vi "数字量输入配置.vi"() -> ()   [LabVIEW 2010] (continued)
              n4462 = local write "单选_第14路"(w132) -> ()
              n4463 = local write "单选_第15路"(w132) -> ()
              n4464 = local write "单选_第16路"(w132) -> ()
              n4465 = local write "单选_第17路"(w132) -> ()
              n4466 = local write "单选_第18路"(w132) -> ()
              n4467 = local write "单选_第19路"(w132) -> ()
              n4468 = local write "单选_第20路"(w132) -> ()
              n4469 = local write "单选_第21路"(w132) -> ()
              n4470 = local write "单选_第22路"(w132) -> ()
              n4471 = local write "单选_第23路"(w132) -> ()
              n4472 = local write "单选_第24路"(w132) -> ()
              n4473 = local write "单选_第25路"(w132) -> ()
              n4474 = local write "单选_第26路"(w132) -> ()
              n4475 = local write "单选_第27路"(w132) -> ()
              n4476 = local write "单选_第28路"(w132) -> ()
              n4477 = local write "单选_第29路"(w132) -> ()
              n4478 = local write "单选_第30路"(w132) -> ()
              n4479 = local write "单选_第31路"(w132) -> ()
              n4480 = local write "单选_第32路"(w132) -> ()
              n4481 = local write "单选_第33路"(w132) -> ()
              n4482 = local write "单选_第34路"(w132) -> ()
              n4483 = local write "单选_第35路"(w132) -> ()
              n4484 = local write "单选_第36路"(w132) -> ()
              n4485 = local write "单选_第37路"(w132) -> ()
              n4486 = local write "单选_第38路"(w132) -> ()
              n4487 = local write "单选_第39路"(w132) -> ()
              n4488 = local write "单选_第40路"(w132) -> ()
              n4489 = local write "单选_第41路"(w132) -> ()
              n4490 = local write "单选_第42路"(w132) -> ()
              n4491 = local write "单选_第43路"(w132) -> ()
              n4492 = local write "单选_第44路"(w132) -> ()
              n4493 = local write "单选_第45路"(w132) -> ()
              n4494 = local write "单选_第46路"(w132) -> ()
              n4495 = local write "单选_第47路"(w132) -> ()
              n4496 = local write "单选_第48路"(w132) -> ()
              n4497 = local write "单选_第49路"(w132) -> ()
              n4498 = local write "单选_第50路"(w132) -> ()
              n4499 = local write "单选_第51路"(w133) -> ()
              n4500 = local write "单选_第52路"(w133) -> ()
              n4501 = local write "单选_第53路"(w133) -> ()
              n4502 = local write "单选_第54路"(w133) -> ()
              n4503 = local write "单选_第55路"(w133) -> ()
              n4504 = local write "单选_第56路"(w133) -> ()
              n4505 = local write "单选_第57路"(w133) -> ()
              n4506 = local write "单选_第58路"(w133) -> ()
              n4507 = local write "单选_第59路"(w133) -> ()
              n4508 = local write "单选_第60路"(w133) -> ()
              n4509 = local write "单选_第61路"(w133) -> ()
              n4510 = local write "单选_第62路"(w133) -> ()
              n4511 = local write "单选_第63路"(w133) -> ()
              n4512 = local write "单选_第64路"(w133) -> ()
              n4513 = local write "单选_第71路"(w133) -> ()
              n4514 = local write "单选_第79路"(w133) -> ()
              n4515 = local write "单选_第65路"(w133) -> ()
              n4516 = local write "单选_第66路"(w133) -> ()
              n4517 = local write "单选_第67路"(w133) -> ()
              n4518 = local write "单选_第68路"(w133) -> ()
              n4519 = local write "单选_第69路"(w133) -> ()
              n4520 = local write "单选_第70路"(w133) -> ()
              n4521 = local write "单选_第72路"(w133) -> ()
              n4522 = local write "单选_第73路"(w133) -> ()
              n4523 = local write "单选_第74路"(w133) -> ()
              n4524 = local write "单选_第75路"(w133) -> ()
              n4525 = local write "单选_第76路"(w133) -> ()
              n4526 = local write "单选_第77路"(w133) -> ()
              n4527 = local write "单选_第78路"(w133) -> ()
              n4528 = local write "单选_第80路"(w133) -> ()
            }
            frame 51 {
              w134 = TRUE
              w135 = FALSE ("单选_第41路")
              n4529 = local write "单选_第1路"(w134) -> ()
              n4530 = local write "单选_第2路"(w134) -> ()
              n4531 = local write "单选_第3路"(w134) -> ()
              n4532 = local write "单选_第4路"(w134) -> ()
              n4533 = local write "单选_第5路"(w134) -> ()
              n4534 = local write "单选_第6路"(w134) -> ()
              n4535 = local write "单选_第7路"(w134) -> ()
              n4536 = local write "单选_第8路"(w134) -> ()
              n4537 = local write "单选_第9路"(w134) -> ()
              n4538 = local write "单选_第10路"(w134) -> ()
              n4539 = local write "单选_第11路"(w134) -> ()
              n4540 = local write "单选_第12路"(w134) -> ()
              n4541 = local write "单选_第13路"(w134) -> ()
              n4542 = local write "单选_第14路"(w134) -> ()
              n4543 = local write "单选_第15路"(w134) -> ()
              n4544 = local write "单选_第16路"(w134) -> ()
              n4545 = local write "单选_第17路"(w134) -> ()
              n4546 = local write "单选_第18路"(w134) -> ()
              n4547 = local write "单选_第19路"(w134) -> ()
              n4548 = local write "单选_第20路"(w134) -> ()
              n4549 = local write "单选_第21路"(w134) -> ()
              n4550 = local write "单选_第22路"(w134) -> ()
              n4551 = local write "单选_第23路"(w134) -> ()
              n4552 = local write "单选_第24路"(w134) -> ()
              n4553 = local write "单选_第25路"(w134) -> ()
              n4554 = local write "单选_第26路"(w134) -> ()
              n4555 = local write "单选_第27路"(w134) -> ()
              n4556 = local write "单选_第28路"(w134) -> ()
              n4557 = local write "单选_第29路"(w134) -> ()
              n4558 = local write "单选_第30路"(w134) -> ()
              n4559 = local write "单选_第31路"(w134) -> ()
              n4560 = local write "单选_第32路"(w134) -> ()
              n4561 = local write "单选_第33路"(w134) -> ()
              n4562 = local write "单选_第34路"(w134) -> ()
              n4563 = local write "单选_第35路"(w134) -> ()
              n4564 = local write "单选_第36路"(w134) -> ()
              n4565 = local write "单选_第37路"(w134) -> ()
              n4566 = local write "单选_第38路"(w134) -> ()
              n4567 = local write "单选_第39路"(w134) -> ()
              n4568 = local write "单选_第40路"(w134) -> ()
              n4569 = local write "单选_第41路"(w134) -> ()
              n4570 = local write "单选_第42路"(w134) -> ()
              n4571 = local write "单选_第43路"(w134) -> ()
              n4572 = local write "单选_第44路"(w134) -> ()
              n4573 = local write "单选_第45路"(w134) -> ()
              n4574 = local write "单选_第46路"(w134) -> ()
              n4575 = local write "单选_第47路"(w134) -> ()
              n4576 = local write "单选_第48路"(w134) -> ()
              n4577 = local write "单选_第49路"(w134) -> ()
              n4578 = local write "单选_第50路"(w134) -> ()
              n4579 = local write "单选_第51路"(w134) -> ()
              n4580 = local write "单选_第52路"(w135) -> ()
              n4581 = local write "单选_第53路"(w135) -> ()
              n4582 = local write "单选_第54路"(w135) -> ()
              n4583 = local write "单选_第55路"(w135) -> ()
              n4584 = local write "单选_第56路"(w135) -> ()
              n4585 = local write "单选_第57路"(w135) -> ()
              n4586 = local write "单选_第58路"(w135) -> ()
              n4587 = local write "单选_第59路"(w135) -> ()
              n4588 = local write "单选_第60路"(w135) -> ()
              n4589 = local write "单选_第61路"(w135) -> ()
              n4590 = local write "单选_第62路"(w135) -> ()
              n4591 = local write "单选_第63路"(w135) -> ()
              n4592 = local write "单选_第64路"(w135) -> ()
              n4593 = local write "单选_第71路"(w135) -> ()
              n4594 = local write "单选_第79路"(w135) -> ()
              n4595 = local write "单选_第65路"(w135) -> ()
              n4596 = local write "单选_第66路"(w135) -> ()
              n4597 = local write "单选_第67路"(w135) -> ()
              n4598 = local write "单选_第68路"(w135) -> ()
              n4599 = local write "单选_第69路"(w135) -> ()
              n4600 = local write "单选_第70路"(w135) -> ()
              n4601 = local write "单选_第72路"(w135) -> ()
              n4602 = local write "单选_第73路"(w135) -> ()
              n4603 = local write "单选_第74路"(w135) -> ()
              n4604 = local write "单选_第75路"(w135) -> ()
              n4605 = local write "单选_第76路"(w135) -> ()
              n4606 = local write "单选_第77路"(w135) -> ()
              n4607 = local write "单选_第78路"(w135) -> ()
              n4608 = local write "单选_第80路"(w135) -> ()
            }
            frame 52 {
              w136 = TRUE
              w137 = FALSE ("单选_第41路")
              n4609 = local write "单选_第1路"(w136) -> ()
              n4610 = local write "单选_第2路"(w136) -> ()
              n4611 = local write "单选_第3路"(w136) -> ()
              n4612 = local write "单选_第4路"(w136) -> ()
              n4613 = local write "单选_第5路"(w136) -> ()
              n4614 = local write "单选_第6路"(w136) -> ()
              n4615 = local write "单选_第7路"(w136) -> ()
              n4616 = local write "单选_第8路"(w136) -> ()
              n4617 = local write "单选_第9路"(w136) -> ()
              n4618 = local write "单选_第10路"(w136) -> ()
              n4619 = local write "单选_第11路"(w136) -> ()
              n4620 = local write "单选_第12路"(w136) -> ()
              n4621 = local write "单选_第13路"(w136) -> ()
              n4622 = local write "单选_第14路"(w136) -> ()
              n4623 = local write "单选_第15路"(w136) -> ()
              n4624 = local write "单选_第16路"(w136) -> ()
              n4625 = local write "单选_第17路"(w136) -> ()
              n4626 = local write "单选_第18路"(w136) -> ()
              n4627 = local write "单选_第19路"(w136) -> ()
              n4628 = local write "单选_第20路"(w136) -> ()
              n4629 = local write "单选_第21路"(w136) -> ()
              n4630 = local write "单选_第22路"(w136) -> ()
              n4631 = local write "单选_第23路"(w136) -> ()
              n4632 = local write "单选_第24路"(w136) -> ()
              n4633 = local write "单选_第25路"(w136) -> ()
              n4634 = local write "单选_第26路"(w136) -> ()
              n4635 = local write "单选_第27路"(w136) -> ()
              n4636 = local write "单选_第28路"(w136) -> ()
              n4637 = local write "单选_第29路"(w136) -> ()
              n4638 = local write "单选_第30路"(w136) -> ()
              n4639 = local write "单选_第31路"(w136) -> ()
              n4640 = local write "单选_第32路"(w136) -> ()
              n4641 = local write "单选_第33路"(w136) -> ()
              n4642 = local write "单选_第34路"(w136) -> ()
              n4643 = local write "单选_第35路"(w136) -> ()
              n4644 = local write "单选_第36路"(w136) -> ()
              n4645 = local write "单选_第37路"(w136) -> ()
              n4646 = local write "单选_第38路"(w136) -> ()
              n4647 = local write "单选_第39路"(w136) -> ()
              n4648 = local write "单选_第40路"(w136) -> ()
              n4649 = local write "单选_第41路"(w136) -> ()
              n4650 = local write "单选_第42路"(w136) -> ()
              n4651 = local write "单选_第43路"(w136) -> ()
              n4652 = local write "单选_第44路"(w136) -> ()
              n4653 = local write "单选_第45路"(w136) -> ()
              n4654 = local write "单选_第46路"(w136) -> ()
              n4655 = local write "单选_第47路"(w136) -> ()
              n4656 = local write "单选_第48路"(w136) -> ()
              n4657 = local write "单选_第49路"(w136) -> ()
              n4658 = local write "单选_第50路"(w136) -> ()
              n4659 = local write "单选_第51路"(w136) -> ()
              n4660 = local write "单选_第52路"(w136) -> ()
              n4661 = local write "单选_第53路"(w137) -> ()
              n4662 = local write "单选_第54路"(w137) -> ()
              n4663 = local write "单选_第55路"(w137) -> ()
              n4664 = local write "单选_第56路"(w137) -> ()
              n4665 = local write "单选_第57路"(w137) -> ()
              n4666 = local write "单选_第58路"(w137) -> ()
              n4667 = local write "单选_第59路"(w137) -> ()
              n4668 = local write "单选_第60路"(w137) -> ()
              n4669 = local write "单选_第61路"(w137) -> ()
              n4670 = local write "单选_第62路"(w137) -> ()
              n4671 = local write "单选_第63路"(w137) -> ()
              n4672 = local write "单选_第64路"(w137) -> ()
              n4673 = local write "单选_第71路"(w137) -> ()
              n4674 = local write "单选_第79路"(w137) -> ()
              n4675 = local write "单选_第65路"(w137) -> ()
              n4676 = local write "单选_第66路"(w137) -> ()
              n4677 = local write "单选_第67路"(w137) -> ()
              n4678 = local write "单选_第68路"(w137) -> ()
              n4679 = local write "单选_第69路"(w137) -> ()
              n4680 = local write "单选_第70路"(w137) -> ()
              n4681 = local write "单选_第72路"(w137) -> ()
              n4682 = local write "单选_第73路"(w137) -> ()
              n4683 = local write "单选_第74路"(w137) -> ()
              n4684 = local write "单选_第75路"(w137) -> ()
              n4685 = local write "单选_第76路"(w137) -> ()
              n4686 = local write "单选_第77路"(w137) -> ()
              n4687 = local write "单选_第78路"(w137) -> ()
              n4688 = local write "单选_第80路"(w137) -> ()
            }
            frame 53 {
              w138 = TRUE
              w139 = FALSE ("单选_第41路")
              n4689 = local write "单选_第1路"(w138) -> ()
              n4690 = local write "单选_第2路"(w138) -> ()
              n4691 = local write "单选_第3路"(w138) -> ()
              n4692 = local write "单选_第4路"(w138) -> ()
              n4693 = local write "单选_第5路"(w138) -> ()
              n4694 = local write "单选_第6路"(w138) -> ()
              n4695 = local write "单选_第7路"(w138) -> ()
              n4696 = local write "单选_第8路"(w138) -> ()
              n4697 = local write "单选_第9路"(w138) -> ()
              n4698 = local write "单选_第10路"(w138) -> ()
              n4699 = local write "单选_第11路"(w138) -> ()
              n4700 = local write "单选_第12路"(w138) -> ()
              n4701 = local write "单选_第13路"(w138) -> ()
              n4702 = local write "单选_第14路"(w138) -> ()
              n4703 = local write "单选_第15路"(w138) -> ()
              n4704 = local write "单选_第16路"(w138) -> ()
              n4705 = local write "单选_第17路"(w138) -> ()
              n4706 = local write "单选_第18路"(w138) -> ()
              n4707 = local write "单选_第19路"(w138) -> ()
              n4708 = local write "单选_第20路"(w138) -> ()
              n4709 = local write "单选_第21路"(w138) -> ()
              n4710 = local write "单选_第22路"(w138) -> ()
              n4711 = local write "单选_第23路"(w138) -> ()
              n4712 = local write "单选_第24路"(w138) -> ()
              n4713 = local write "单选_第25路"(w138) -> ()
              n4714 = local write "单选_第26路"(w138) -> ()
              n4715 = local write "单选_第27路"(w138) -> ()
              n4716 = local write "单选_第28路"(w138) -> ()
              n4717 = local write "单选_第29路"(w138) -> ()
              n4718 = local write "单选_第30路"(w138) -> ()
              n4719 = local write "单选_第31路"(w138) -> ()
              n4720 = local write "单选_第32路"(w138) -> ()
              n4721 = local write "单选_第33路"(w138) -> ()
              n4722 = local write "单选_第34路"(w138) -> ()
              n4723 = local write "单选_第35路"(w138) -> ()
              n4724 = local write "单选_第36路"(w138) -> ()
              n4725 = local write "单选_第37路"(w138) -> ()
              n4726 = local write "单选_第38路"(w138) -> ()
              n4727 = local write "单选_第39路"(w138) -> ()
              n4728 = local write "单选_第40路"(w138) -> ()
              n4729 = local write "单选_第41路"(w138) -> ()
              n4730 = local write "单选_第42路"(w138) -> ()
              n4731 = local write "单选_第43路"(w138) -> ()
              n4732 = local write "单选_第44路"(w138) -> ()
              n4733 = local write "单选_第45路"(w138) -> ()
              n4734 = local write "单选_第46路"(w138) -> ()
              n4735 = local write "单选_第47路"(w138) -> ()
              n4736 = local write "单选_第48路"(w138) -> ()
              n4737 = local write "单选_第49路"(w138) -> ()
              n4738 = local write "单选_第50路"(w138) -> ()
              n4739 = local write "单选_第51路"(w138) -> ()
              n4740 = local write "单选_第52路"(w138) -> ()
              n4741 = local write "单选_第53路"(w138) -> ()
              n4742 = local write "单选_第54路"(w139) -> ()
              n4743 = local write "单选_第55路"(w139) -> ()
              n4744 = local write "单选_第56路"(w139) -> ()
              n4745 = local write "单选_第57路"(w139) -> ()
              n4746 = local write "单选_第58路"(w139) -> ()
              n4747 = local write "单选_第59路"(w139) -> ()
              n4748 = local write "单选_第60路"(w139) -> ()
              n4749 = local write "单选_第61路"(w139) -> ()
              n4750 = local write "单选_第62路"(w139) -> ()
              n4751 = local write "单选_第63路"(w139) -> ()
              n4752 = local write "单选_第64路"(w139) -> ()
              n4753 = local write "单选_第71路"(w139) -> ()
              n4754 = local write "单选_第79路"(w139) -> ()
              n4755 = local write "单选_第65路"(w139) -> ()
              n4756 = local write "单选_第66路"(w139) -> ()
              n4757 = local write "单选_第67路"(w139) -> ()
              n4758 = local write "单选_第68路"(w139) -> ()
              n4759 = local write "单选_第69路"(w139) -> ()
              n4760 = local write "单选_第70路"(w139) -> ()
              n4761 = local write "单选_第72路"(w139) -> ()
              n4762 = local write "单选_第73路"(w139) -> ()
              n4763 = local write "单选_第74路"(w139) -> ()
              n4764 = local write "单选_第75路"(w139) -> ()
              n4765 = local write "单选_第76路"(w139) -> ()
              n4766 = local write "单选_第77路"(w139) -> ()
              n4767 = local write "单选_第78路"(w139) -> ()
              n4768 = local write "单选_第80路"(w139) -> ()
            }
            frame 54 {
              w140 = TRUE
              w141 = FALSE ("单选_第41路")
              n4769 = local write "单选_第1路"(w140) -> ()
              n4770 = local write "单选_第2路"(w140) -> ()
              n4771 = local write "单选_第3路"(w140) -> ()
              n4772 = local write "单选_第4路"(w140) -> ()
              n4773 = local write "单选_第5路"(w140) -> ()
              n4774 = local write "单选_第6路"(w140) -> ()
              n4775 = local write "单选_第7路"(w140) -> ()
              n4776 = local write "单选_第8路"(w140) -> ()
              n4777 = local write "单选_第9路"(w140) -> ()
              n4778 = local write "单选_第10路"(w140) -> ()
              n4779 = local write "单选_第11路"(w140) -> ()
              n4780 = local write "单选_第12路"(w140) -> ()
              n4781 = local write "单选_第13路"(w140) -> ()
              n4782 = local write "单选_第14路"(w140) -> ()
              n4783 = local write "单选_第15路"(w140) -> ()
              n4784 = local write "单选_第16路"(w140) -> ()
              n4785 = local write "单选_第17路"(w140) -> ()
              n4786 = local write "单选_第18路"(w140) -> ()
              n4787 = local write "单选_第19路"(w140) -> ()
              n4788 = local write "单选_第20路"(w140) -> ()
              n4789 = local write "单选_第21路"(w140) -> ()
              n4790 = local write "单选_第22路"(w140) -> ()
              n4791 = local write "单选_第23路"(w140) -> ()
              n4792 = local write "单选_第24路"(w140) -> ()
              n4793 = local write "单选_第25路"(w140) -> ()
              n4794 = local write "单选_第26路"(w140) -> ()
              n4795 = local write "单选_第27路"(w140) -> ()
              n4796 = local write "单选_第28路"(w140) -> ()
              n4797 = local write "单选_第29路"(w140) -> ()
              n4798 = local write "单选_第30路"(w140) -> ()
              n4799 = local write "单选_第31路"(w140) -> ()
              n4800 = local write "单选_第32路"(w140) -> ()
              n4801 = local write "单选_第33路"(w140) -> ()
              n4802 = local write "单选_第34路"(w140) -> ()
              n4803 = local write "单选_第35路"(w140) -> ()
              n4804 = local write "单选_第36路"(w140) -> ()
              n4805 = local write "单选_第37路"(w140) -> ()
              n4806 = local write "单选_第38路"(w140) -> ()
              n4807 = local write "单选_第39路"(w140) -> ()
              n4808 = local write "单选_第40路"(w140) -> ()
              n4809 = local write "单选_第41路"(w140) -> ()
              n4810 = local write "单选_第42路"(w140) -> ()
              n4811 = local write "单选_第43路"(w140) -> ()
              n4812 = local write "单选_第44路"(w140) -> ()
              n4813 = local write "单选_第45路"(w140) -> ()
              n4814 = local write "单选_第46路"(w140) -> ()
              n4815 = local write "单选_第47路"(w140) -> ()
              n4816 = local write "单选_第48路"(w140) -> ()
              n4817 = local write "单选_第49路"(w140) -> ()
              n4818 = local write "单选_第50路"(w140) -> ()
              n4819 = local write "单选_第51路"(w140) -> ()
              n4820 = local write "单选_第52路"(w140) -> ()
              n4821 = local write "单选_第53路"(w140) -> ()
              n4822 = local write "单选_第54路"(w140) -> ()
              n4823 = local write "单选_第55路"(w141) -> ()
              n4824 = local write "单选_第56路"(w141) -> ()
              n4825 = local write "单选_第57路"(w141) -> ()
              n4826 = local write "单选_第58路"(w141) -> ()
              n4827 = local write "单选_第59路"(w141) -> ()
              n4828 = local write "单选_第60路"(w141) -> ()
              n4829 = local write "单选_第61路"(w141) -> ()
              n4830 = local write "单选_第62路"(w141) -> ()
              n4831 = local write "单选_第63路"(w141) -> ()
              n4832 = local write "单选_第64路"(w141) -> ()
              n4833 = local write "单选_第71路"(w141) -> ()
              n4834 = local write "单选_第79路"(w141) -> ()
              n4835 = local write "单选_第65路"(w141) -> ()
              n4836 = local write "单选_第66路"(w141) -> ()
              n4837 = local write "单选_第67路"(w141) -> ()
              n4838 = local write "单选_第68路"(w141) -> ()
              n4839 = local write "单选_第69路"(w141) -> ()
              n4840 = local write "单选_第70路"(w141) -> ()
              n4841 = local write "单选_第72路"(w141) -> ()
              n4842 = local write "单选_第73路"(w141) -> ()
              n4843 = local write "单选_第74路"(w141) -> ()
              n4844 = local write "单选_第75路"(w141) -> ()
              n4845 = local write "单选_第76路"(w141) -> ()
              n4846 = local write "单选_第77路"(w141) -> ()
              n4847 = local write "单选_第78路"(w141) -> ()
              n4848 = local write "单选_第80路"(w141) -> ()
            }
            frame 55 {
              w142 = TRUE
              w143 = FALSE ("单选_第41路")
              n4849 = local write "单选_第1路"(w142) -> ()
              n4850 = local write "单选_第2路"(w142) -> ()
              n4851 = local write "单选_第3路"(w142) -> ()
              n4852 = local write "单选_第4路"(w142) -> ()
              n4853 = local write "单选_第5路"(w142) -> ()
              n4854 = local write "单选_第6路"(w142) -> ()
              n4855 = local write "单选_第7路"(w142) -> ()
              n4856 = local write "单选_第8路"(w142) -> ()
              n4857 = local write "单选_第9路"(w142) -> ()
              n4858 = local write "单选_第10路"(w142) -> ()
              n4859 = local write "单选_第11路"(w142) -> ()
              n4860 = local write "单选_第12路"(w142) -> ()
              n4861 = local write "单选_第13路"(w142) -> ()
              n4862 = local write "单选_第14路"(w142) -> ()
              n4863 = local write "单选_第15路"(w142) -> ()
              n4864 = local write "单选_第16路"(w142) -> ()
              n4865 = local write "单选_第17路"(w142) -> ()
              n4866 = local write "单选_第18路"(w142) -> ()
              n4867 = local write "单选_第19路"(w142) -> ()
              n4868 = local write "单选_第20路"(w142) -> ()
              n4869 = local write "单选_第21路"(w142) -> ()
              n4870 = local write "单选_第22路"(w142) -> ()
              n4871 = local write "单选_第23路"(w142) -> ()
              n4872 = local write "单选_第24路"(w142) -> ()
              n4873 = local write "单选_第25路"(w142) -> ()
              n4874 = local write "单选_第26路"(w142) -> ()
              n4875 = local write "单选_第27路"(w142) -> ()
              n4876 = local write "单选_第28路"(w142) -> ()
              n4877 = local write "单选_第29路"(w142) -> ()
              n4878 = local write "单选_第30路"(w142) -> ()
              n4879 = local write "单选_第31路"(w142) -> ()
              n4880 = local write "单选_第32路"(w142) -> ()
              n4881 = local write "单选_第33路"(w142) -> ()
              n4882 = local write "单选_第34路"(w142) -> ()
              n4883 = local write "单选_第35路"(w142) -> ()
              n4884 = local write "单选_第36路"(w142) -> ()
              n4885 = local write "单选_第37路"(w142) -> ()
              n4886 = local write "单选_第38路"(w142) -> ()
              n4887 = local write "单选_第39路"(w142) -> ()
              n4888 = local write "单选_第40路"(w142) -> ()
              n4889 = local write "单选_第41路"(w142) -> ()
              n4890 = local write "单选_第42路"(w142) -> ()
              n4891 = local write "单选_第43路"(w142) -> ()
              n4892 = local write "单选_第44路"(w142) -> ()
              n4893 = local write "单选_第45路"(w142) -> ()
              n4894 = local write "单选_第46路"(w142) -> ()
              n4895 = local write "单选_第47路"(w142) -> ()
              n4896 = local write "单选_第48路"(w142) -> ()
              n4897 = local write "单选_第49路"(w142) -> ()
              n4898 = local write "单选_第50路"(w142) -> ()
              n4899 = local write "单选_第51路"(w142) -> ()
              n4900 = local write "单选_第52路"(w142) -> ()
              n4901 = local write "单选_第53路"(w142) -> ()
              n4902 = local write "单选_第54路"(w142) -> ()
              n4903 = local write "单选_第55路"(w142) -> ()
              n4904 = local write "单选_第56路"(w143) -> ()
              n4905 = local write "单选_第57路"(w143) -> ()
              n4906 = local write "单选_第58路"(w143) -> ()
              n4907 = local write "单选_第59路"(w143) -> ()
              n4908 = local write "单选_第60路"(w143) -> ()
              n4909 = local write "单选_第61路"(w143) -> ()
              n4910 = local write "单选_第62路"(w143) -> ()
              n4911 = local write "单选_第63路"(w143) -> ()
              n4912 = local write "单选_第64路"(w143) -> ()
              n4913 = local write "单选_第71路"(w143) -> ()
              n4914 = local write "单选_第79路"(w143) -> ()
              n4915 = local write "单选_第65路"(w143) -> ()
              n4916 = local write "单选_第66路"(w143) -> ()
              n4917 = local write "单选_第67路"(w143) -> ()
              n4918 = local write "单选_第68路"(w143) -> ()
              n4919 = local write "单选_第69路"(w143) -> ()
              n4920 = local write "单选_第70路"(w143) -> ()
              n4921 = local write "单选_第72路"(w143) -> ()
              n4922 = local write "单选_第73路"(w143) -> ()
              n4923 = local write "单选_第74路"(w143) -> ()
              n4924 = local write "单选_第75路"(w143) -> ()
              n4925 = local write "单选_第76路"(w143) -> ()
              n4926 = local write "单选_第77路"(w143) -> ()
              n4927 = local write "单选_第78路"(w143) -> ()
              n4928 = local write "单选_第80路"(w143) -> ()
            }
            frame 56 {
              w144 = TRUE
              w145 = FALSE ("单选_第41路")
              n4929 = local write "单选_第1路"(w144) -> ()
              n4930 = local write "单选_第2路"(w144) -> ()
              n4931 = local write "单选_第3路"(w144) -> ()
              n4932 = local write "单选_第4路"(w144) -> ()
              n4933 = local write "单选_第5路"(w144) -> ()
              n4934 = local write "单选_第6路"(w144) -> ()
              n4935 = local write "单选_第7路"(w144) -> ()
              n4936 = local write "单选_第8路"(w144) -> ()
              n4937 = local write "单选_第9路"(w144) -> ()
              n4938 = local write "单选_第10路"(w144) -> ()
              n4939 = local write "单选_第11路"(w144) -> ()
              n4940 = local write "单选_第12路"(w144) -> ()
              n4941 = local write "单选_第13路"(w144) -> ()
              n4942 = local write "单选_第14路"(w144) -> ()
              n4943 = local write "单选_第15路"(w144) -> ()
              n4944 = local write "单选_第16路"(w144) -> ()
              n4945 = local write "单选_第17路"(w144) -> ()
              n4946 = local write "单选_第18路"(w144) -> ()
              n4947 = local write "单选_第19路"(w144) -> ()
              n4948 = local write "单选_第20路"(w144) -> ()
              n4949 = local write "单选_第21路"(w144) -> ()
              n4950 = local write "单选_第22路"(w144) -> ()
              n4951 = local write "单选_第23路"(w144) -> ()
              n4952 = local write "单选_第24路"(w144) -> ()
              n4953 = local write "单选_第25路"(w144) -> ()
              n4954 = local write "单选_第26路"(w144) -> ()
              n4955 = local write "单选_第27路"(w144) -> ()
              n4956 = local write "单选_第28路"(w144) -> ()
              n4957 = local write "单选_第29路"(w144) -> ()
              n4958 = local write "单选_第30路"(w144) -> ()
              n4959 = local write "单选_第31路"(w144) -> ()
              n4960 = local write "单选_第32路"(w144) -> ()
              n4961 = local write "单选_第33路"(w144) -> ()
              n4962 = local write "单选_第34路"(w144) -> ()
              n4963 = local write "单选_第35路"(w144) -> ()
              n4964 = local write "单选_第36路"(w144) -> ()
              n4965 = local write "单选_第37路"(w144) -> ()
              n4966 = local write "单选_第38路"(w144) -> ()
              n4967 = local write "单选_第39路"(w144) -> ()
              n4968 = local write "单选_第40路"(w144) -> ()
              n4969 = local write "单选_第41路"(w144) -> ()
              n4970 = local write "单选_第42路"(w144) -> ()
              n4971 = local write "单选_第43路"(w144) -> ()
              n4972 = local write "单选_第44路"(w144) -> ()
              n4973 = local write "单选_第45路"(w144) -> ()
              n4974 = local write "单选_第46路"(w144) -> ()
              n4975 = local write "单选_第47路"(w144) -> ()
              n4976 = local write "单选_第48路"(w144) -> ()
              n4977 = local write "单选_第49路"(w144) -> ()
              n4978 = local write "单选_第50路"(w144) -> ()
              n4979 = local write "单选_第51路"(w144) -> ()
              n4980 = local write "单选_第52路"(w144) -> ()
              n4981 = local write "单选_第53路"(w144) -> ()
              n4982 = local write "单选_第54路"(w144) -> ()
              n4983 = local write "单选_第55路"(w144) -> ()
              n4984 = local write "单选_第56路"(w144) -> ()
              n4985 = local write "单选_第57路"(w145) -> ()
              n4986 = local write "单选_第58路"(w145) -> ()
              n4987 = local write "单选_第59路"(w145) -> ()
              n4988 = local write "单选_第60路"(w145) -> ()
              n4989 = local write "单选_第61路"(w145) -> ()
              n4990 = local write "单选_第62路"(w145) -> ()
              n4991 = local write "单选_第63路"(w145) -> ()
              n4992 = local write "单选_第64路"(w145) -> ()
              n4993 = local write "单选_第71路"(w145) -> ()
              n4994 = local write "单选_第79路"(w145) -> ()
              n4995 = local write "单选_第65路"(w145) -> ()
              n4996 = local write "单选_第66路"(w145) -> ()
              n4997 = local write "单选_第67路"(w145) -> ()
              n4998 = local write "单选_第68路"(w145) -> ()
              n4999 = local write "单选_第69路"(w145) -> ()
              n5000 = local write "单选_第70路"(w145) -> ()
              n5001 = local write "单选_第72路"(w145) -> ()
              n5002 = local write "单选_第73路"(w145) -> ()
              n5003 = local write "单选_第74路"(w145) -> ()
              n5004 = local write "单选_第75路"(w145) -> ()
              n5005 = local write "单选_第76路"(w145) -> ()
              n5006 = local write "单选_第77路"(w145) -> ()
              n5007 = local write "单选_第78路"(w145) -> ()
              n5008 = local write "单选_第80路"(w145) -> ()
            }
            frame 57 {
              w146 = TRUE
              w147 = FALSE ("单选_第41路")
              n5009 = local write "单选_第1路"(w146) -> ()
              n5010 = local write "单选_第2路"(w146) -> ()
              n5011 = local write "单选_第3路"(w146) -> ()
              n5012 = local write "单选_第4路"(w146) -> ()
              n5013 = local write "单选_第5路"(w146) -> ()
              n5014 = local write "单选_第6路"(w146) -> ()
              n5015 = local write "单选_第7路"(w146) -> ()
              n5016 = local write "单选_第8路"(w146) -> ()
              n5017 = local write "单选_第9路"(w146) -> ()
              n5018 = local write "单选_第10路"(w146) -> ()
              n5019 = local write "单选_第11路"(w146) -> ()
              n5020 = local write "单选_第12路"(w146) -> ()
              n5021 = local write "单选_第13路"(w146) -> ()
              n5022 = local write "单选_第14路"(w146) -> ()
              n5023 = local write "单选_第15路"(w146) -> ()
              n5024 = local write "单选_第16路"(w146) -> ()
              n5025 = local write "单选_第17路"(w146) -> ()
              n5026 = local write "单选_第18路"(w146) -> ()
              n5027 = local write "单选_第19路"(w146) -> ()
              n5028 = local write "单选_第20路"(w146) -> ()
              n5029 = local write "单选_第21路"(w146) -> ()
              n5030 = local write "单选_第22路"(w146) -> ()
              n5031 = local write "单选_第23路"(w146) -> ()
              n5032 = local write "单选_第24路"(w146) -> ()
              n5033 = local write "单选_第25路"(w146) -> ()
              n5034 = local write "单选_第26路"(w146) -> ()
              n5035 = local write "单选_第27路"(w146) -> ()
              n5036 = local write "单选_第28路"(w146) -> ()
              n5037 = local write "单选_第29路"(w146) -> ()
              n5038 = local write "单选_第30路"(w146) -> ()
              n5039 = local write "单选_第31路"(w146) -> ()
              n5040 = local write "单选_第32路"(w146) -> ()
              n5041 = local write "单选_第33路"(w146) -> ()
              n5042 = local write "单选_第34路"(w146) -> ()
              n5043 = local write "单选_第35路"(w146) -> ()
              n5044 = local write "单选_第36路"(w146) -> ()
              n5045 = local write "单选_第37路"(w146) -> ()
              n5046 = local write "单选_第38路"(w146) -> ()
              n5047 = local write "单选_第39路"(w146) -> ()
              n5048 = local write "单选_第40路"(w146) -> ()
              n5049 = local write "单选_第41路"(w146) -> ()
              n5050 = local write "单选_第42路"(w146) -> ()
              n5051 = local write "单选_第43路"(w146) -> ()
              n5052 = local write "单选_第44路"(w146) -> ()
              n5053 = local write "单选_第45路"(w146) -> ()
              n5054 = local write "单选_第46路"(w146) -> ()
              n5055 = local write "单选_第47路"(w146) -> ()
              n5056 = local write "单选_第48路"(w146) -> ()
              n5057 = local write "单选_第49路"(w146) -> ()
              n5058 = local write "单选_第50路"(w146) -> ()
              n5059 = local write "单选_第51路"(w146) -> ()
              n5060 = local write "单选_第52路"(w146) -> ()
              n5061 = local write "单选_第53路"(w146) -> ()
              n5062 = local write "单选_第54路"(w146) -> ()
              n5063 = local write "单选_第55路"(w146) -> ()
              n5064 = local write "单选_第56路"(w146) -> ()
              n5065 = local write "单选_第57路"(w146) -> ()
              n5066 = local write "单选_第58路"(w147) -> ()
              n5067 = local write "单选_第59路"(w147) -> ()
              n5068 = local write "单选_第60路"(w147) -> ()
              n5069 = local write "单选_第61路"(w147) -> ()
              n5070 = local write "单选_第62路"(w147) -> ()
              n5071 = local write "单选_第63路"(w147) -> ()
              n5072 = local write "单选_第64路"(w147) -> ()
              n5073 = local write "单选_第71路"(w147) -> ()
              n5074 = local write "单选_第79路"(w147) -> ()
              n5075 = local write "单选_第65路"(w147) -> ()
              n5076 = local write "单选_第66路"(w147) -> ()
              n5077 = local write "单选_第67路"(w147) -> ()
              n5078 = local write "单选_第68路"(w147) -> ()
              n5079 = local write "单选_第69路"(w147) -> ()
              n5080 = local write "单选_第70路"(w147) -> ()
              n5081 = local write "单选_第72路"(w147) -> ()
              n5082 = local write "单选_第73路"(w147) -> ()
              n5083 = local write "单选_第74路"(w147) -> ()
              n5084 = local write "单选_第75路"(w147) -> ()
              n5085 = local write "单选_第76路"(w147) -> ()
              n5086 = local write "单选_第77路"(w147) -> ()
              n5087 = local write "单选_第78路"(w147) -> ()
              n5088 = local write "单选_第80路"(w147) -> ()
            }
            frame 58 {
              w148 = TRUE
              w149 = FALSE ("单选_第41路")
              n5089 = local write "单选_第1路"(w148) -> ()
              n5090 = local write "单选_第2路"(w148) -> ()
              n5091 = local write "单选_第3路"(w148) -> ()
              n5092 = local write "单选_第4路"(w148) -> ()
              n5093 = local write "单选_第5路"(w148) -> ()
              n5094 = local write "单选_第6路"(w148) -> ()
              n5095 = local write "单选_第7路"(w148) -> ()
              n5096 = local write "单选_第8路"(w148) -> ()
              n5097 = local write "单选_第9路"(w148) -> ()
              n5098 = local write "单选_第10路"(w148) -> ()
              n5099 = local write "单选_第11路"(w148) -> ()
              n5100 = local write "单选_第12路"(w148) -> ()
              n5101 = local write "单选_第13路"(w148) -> ()
              n5102 = local write "单选_第14路"(w148) -> ()
              n5103 = local write "单选_第15路"(w148) -> ()
              n5104 = local write "单选_第16路"(w148) -> ()
              n5105 = local write "单选_第17路"(w148) -> ()
              n5106 = local write "单选_第18路"(w148) -> ()
              n5107 = local write "单选_第19路"(w148) -> ()
              n5108 = local write "单选_第20路"(w148) -> ()
              n5109 = local write "单选_第21路"(w148) -> ()
              n5110 = local write "单选_第22路"(w148) -> ()
              n5111 = local write "单选_第23路"(w148) -> ()
              n5112 = local write "单选_第24路"(w148) -> ()
              n5113 = local write "单选_第25路"(w148) -> ()
              n5114 = local write "单选_第26路"(w148) -> ()
              n5115 = local write "单选_第27路"(w148) -> ()
              n5116 = local write "单选_第28路"(w148) -> ()
              n5117 = local write "单选_第29路"(w148) -> ()
              n5118 = local write "单选_第30路"(w148) -> ()
              n5119 = local write "单选_第31路"(w148) -> ()
              n5120 = local write "单选_第32路"(w148) -> ()
              n5121 = local write "单选_第33路"(w148) -> ()
              n5122 = local write "单选_第34路"(w148) -> ()
              n5123 = local write "单选_第35路"(w148) -> ()
              n5124 = local write "单选_第36路"(w148) -> ()
              n5125 = local write "单选_第37路"(w148) -> ()
              n5126 = local write "单选_第38路"(w148) -> ()
              n5127 = local write "单选_第39路"(w148) -> ()
              n5128 = local write "单选_第40路"(w148) -> ()
              n5129 = local write "单选_第41路"(w148) -> ()
              n5130 = local write "单选_第42路"(w148) -> ()
              n5131 = local write "单选_第43路"(w148) -> ()
              n5132 = local write "单选_第44路"(w148) -> ()
              n5133 = local write "单选_第45路"(w148) -> ()
              n5134 = local write "单选_第46路"(w148) -> ()
              n5135 = local write "单选_第47路"(w148) -> ()
              n5136 = local write "单选_第48路"(w148) -> ()
              n5137 = local write "单选_第49路"(w148) -> ()
              n5138 = local write "单选_第50路"(w148) -> ()
              n5139 = local write "单选_第51路"(w148) -> ()
              n5140 = local write "单选_第52路"(w148) -> ()
              n5141 = local write "单选_第53路"(w148) -> ()
              n5142 = local write "单选_第54路"(w148) -> ()
              n5143 = local write "单选_第55路"(w148) -> ()
              n5144 = local write "单选_第56路"(w148) -> ()
              n5145 = local write "单选_第57路"(w148) -> ()
              n5146 = local write "单选_第58路"(w148) -> ()
              n5147 = local write "单选_第59路"(w149) -> ()
              n5148 = local write "单选_第60路"(w149) -> ()
              n5149 = local write "单选_第61路"(w149) -> ()
              n5150 = local write "单选_第62路"(w149) -> ()
              n5151 = local write "单选_第63路"(w149) -> ()
              n5152 = local write "单选_第64路"(w149) -> ()
              n5153 = local write "单选_第71路"(w149) -> ()
              n5154 = local write "单选_第79路"(w149) -> ()
              n5155 = local write "单选_第65路"(w149) -> ()
              n5156 = local write "单选_第66路"(w149) -> ()
              n5157 = local write "单选_第67路"(w149) -> ()
              n5158 = local write "单选_第68路"(w149) -> ()
              n5159 = local write "单选_第69路"(w149) -> ()
              n5160 = local write "单选_第70路"(w149) -> ()
              n5161 = local write "单选_第72路"(w149) -> ()
              n5162 = local write "单选_第73路"(w149) -> ()
              n5163 = local write "单选_第74路"(w149) -> ()
              n5164 = local write "单选_第75路"(w149) -> ()
              n5165 = local write "单选_第76路"(w149) -> ()
              n5166 = local write "单选_第77路"(w149) -> ()
              n5167 = local write "单选_第78路"(w149) -> ()
              n5168 = local write "单选_第80路"(w149) -> ()
            }
            frame 59 {
              w150 = TRUE
              w151 = FALSE ("单选_第41路")
              n5169 = local write "单选_第1路"(w150) -> ()
              n5170 = local write "单选_第2路"(w150) -> ()
              n5171 = local write "单选_第3路"(w150) -> ()
              n5172 = local write "单选_第4路"(w150) -> ()
              n5173 = local write "单选_第5路"(w150) -> ()
              n5174 = local write "单选_第6路"(w150) -> ()
              n5175 = local write "单选_第7路"(w150) -> ()
              n5176 = local write "单选_第8路"(w150) -> ()
              n5177 = local write "单选_第9路"(w150) -> ()
              n5178 = local write "单选_第10路"(w150) -> ()
              n5179 = local write "单选_第11路"(w150) -> ()
              n5180 = local write "单选_第12路"(w150) -> ()
              n5181 = local write "单选_第13路"(w150) -> ()
              n5182 = local write "单选_第14路"(w150) -> ()
              n5183 = local write "单选_第15路"(w150) -> ()
              n5184 = local write "单选_第16路"(w150) -> ()
              n5185 = local write "单选_第17路"(w150) -> ()
              n5186 = local write "单选_第18路"(w150) -> ()
              n5187 = local write "单选_第19路"(w150) -> ()
              n5188 = local write "单选_第20路"(w150) -> ()
              n5189 = local write "单选_第21路"(w150) -> ()
              n5190 = local write "单选_第22路"(w150) -> ()
              n5191 = local write "单选_第23路"(w150) -> ()
              n5192 = local write "单选_第24路"(w150) -> ()
              n5193 = local write "单选_第25路"(w150) -> ()
              n5194 = local write "单选_第26路"(w150) -> ()
              n5195 = local write "单选_第27路"(w150) -> ()
              n5196 = local write "单选_第28路"(w150) -> ()
              n5197 = local write "单选_第29路"(w150) -> ()
              n5198 = local write "单选_第30路"(w150) -> ()
              n5199 = local write "单选_第31路"(w150) -> ()
              n5200 = local write "单选_第32路"(w150) -> ()
              n5201 = local write "单选_第33路"(w150) -> ()
              n5202 = local write "单选_第34路"(w150) -> ()
              n5203 = local write "单选_第35路"(w150) -> ()
              n5204 = local write "单选_第36路"(w150) -> ()
              n5205 = local write "单选_第37路"(w150) -> ()
              n5206 = local write "单选_第38路"(w150) -> ()
              n5207 = local write "单选_第39路"(w150) -> ()
              n5208 = local write "单选_第40路"(w150) -> ()
              n5209 = local write "单选_第41路"(w150) -> ()
              n5210 = local write "单选_第42路"(w150) -> ()
              n5211 = local write "单选_第43路"(w150) -> ()
              n5212 = local write "单选_第44路"(w150) -> ()
              n5213 = local write "单选_第45路"(w150) -> ()
              n5214 = local write "单选_第46路"(w150) -> ()
              n5215 = local write "单选_第47路"(w150) -> ()
              n5216 = local write "单选_第48路"(w150) -> ()
              n5217 = local write "单选_第49路"(w150) -> ()
              n5218 = local write "单选_第50路"(w150) -> ()
              n5219 = local write "单选_第51路"(w150) -> ()
              n5220 = local write "单选_第52路"(w150) -> ()
              n5221 = local write "单选_第53路"(w150) -> ()
              n5222 = local write "单选_第54路"(w150) -> ()
              n5223 = local write "单选_第55路"(w150) -> ()
              n5224 = local write "单选_第56路"(w150) -> ()
              n5225 = local write "单选_第57路"(w150) -> ()
              n5226 = local write "单选_第58路"(w150) -> ()
              n5227 = local write "单选_第59路"(w150) -> ()
              n5228 = local write "单选_第60路"(w151) -> ()
              n5229 = local write "单选_第61路"(w151) -> ()
              n5230 = local write "单选_第62路"(w151) -> ()
              n5231 = local write "单选_第63路"(w151) -> ()
              n5232 = local write "单选_第64路"(w151) -> ()
              n5233 = local write "单选_第71路"(w151) -> ()
              n5234 = local write "单选_第79路"(w151) -> ()
              n5235 = local write "单选_第65路"(w151) -> ()
              n5236 = local write "单选_第66路"(w151) -> ()
              n5237 = local write "单选_第67路"(w151) -> ()
              n5238 = local write "单选_第68路"(w151) -> ()
              n5239 = local write "单选_第69路"(w151) -> ()
              n5240 = local write "单选_第70路"(w151) -> ()
              n5241 = local write "单选_第72路"(w151) -> ()
              n5242 = local write "单选_第73路"(w151) -> ()
              n5243 = local write "单选_第74路"(w151) -> ()
              n5244 = local write "单选_第75路"(w151) -> ()
              n5245 = local write "单选_第76路"(w151) -> ()
              n5246 = local write "单选_第77路"(w151) -> ()
              n5247 = local write "单选_第78路"(w151) -> ()
              n5248 = local write "单选_第80路"(w151) -> ()
            }
            frame 60 {
              w152 = TRUE
              w153 = FALSE ("单选_第41路")
              n5249 = local write "单选_第1路"(w152) -> ()
              n5250 = local write "单选_第2路"(w152) -> ()
              n5251 = local write "单选_第3路"(w152) -> ()
              n5252 = local write "单选_第4路"(w152) -> ()
              n5253 = local write "单选_第5路"(w152) -> ()
              n5254 = local write "单选_第6路"(w152) -> ()
              n5255 = local write "单选_第7路"(w152) -> ()
              n5256 = local write "单选_第8路"(w152) -> ()
              n5257 = local write "单选_第9路"(w152) -> ()
              n5258 = local write "单选_第10路"(w152) -> ()
              n5259 = local write "单选_第11路"(w152) -> ()
              n5260 = local write "单选_第12路"(w152) -> ()
              n5261 = local write "单选_第13路"(w152) -> ()
              n5262 = local write "单选_第14路"(w152) -> ()
              n5263 = local write "单选_第15路"(w152) -> ()
              n5264 = local write "单选_第16路"(w152) -> ()
              n5265 = local write "单选_第17路"(w152) -> ()
              n5266 = local write "单选_第18路"(w152) -> ()
              n5267 = local write "单选_第19路"(w152) -> ()
              n5268 = local write "单选_第20路"(w152) -> ()
              n5269 = local write "单选_第21路"(w152) -> ()
              n5270 = local write "单选_第22路"(w152) -> ()
              n5271 = local write "单选_第23路"(w152) -> ()
              n5272 = local write "单选_第24路"(w152) -> ()
              n5273 = local write "单选_第25路"(w152) -> ()
              n5274 = local write "单选_第26路"(w152) -> ()
              n5275 = local write "单选_第27路"(w152) -> ()
              n5276 = local write "单选_第28路"(w152) -> ()
              n5277 = local write "单选_第29路"(w152) -> ()
              n5278 = local write "单选_第30路"(w152) -> ()
              n5279 = local write "单选_第31路"(w152) -> ()
              n5280 = local write "单选_第32路"(w152) -> ()
              n5281 = local write "单选_第33路"(w152) -> ()
              n5282 = local write "单选_第34路"(w152) -> ()
              n5283 = local write "单选_第35路"(w152) -> ()
              n5284 = local write "单选_第36路"(w152) -> ()
              n5285 = local write "单选_第37路"(w152) -> ()
              n5286 = local write "单选_第38路"(w152) -> ()
              n5287 = local write "单选_第39路"(w152) -> ()
              n5288 = local write "单选_第40路"(w152) -> ()
              n5289 = local write "单选_第41路"(w152) -> ()
              n5290 = local write "单选_第42路"(w152) -> ()
              n5291 = local write "单选_第43路"(w152) -> ()
              n5292 = local write "单选_第44路"(w152) -> ()
              n5293 = local write "单选_第45路"(w152) -> ()
              n5294 = local write "单选_第46路"(w152) -> ()
              n5295 = local write "单选_第47路"(w152) -> ()
              n5296 = local write "单选_第48路"(w152) -> ()
              n5297 = local write "单选_第49路"(w152) -> ()
              n5298 = local write "单选_第50路"(w152) -> ()
              n5299 = local write "单选_第51路"(w152) -> ()
              n5300 = local write "单选_第52路"(w152) -> ()
              n5301 = local write "单选_第53路"(w152) -> ()
              n5302 = local write "单选_第54路"(w152) -> ()
              n5303 = local write "单选_第55路"(w152) -> ()
              n5304 = local write "单选_第56路"(w152) -> ()
              n5305 = local write "单选_第57路"(w152) -> ()
              n5306 = local write "单选_第58路"(w152) -> ()
              n5307 = local write "单选_第59路"(w152) -> ()
              n5308 = local write "单选_第60路"(w152) -> ()
              n5309 = local write "单选_第61路"(w153) -> ()
              n5310 = local write "单选_第62路"(w153) -> ()
              n5311 = local write "单选_第63路"(w153) -> ()
              n5312 = local write "单选_第64路"(w153) -> ()
              n5313 = local write "单选_第71路"(w153) -> ()
              n5314 = local write "单选_第79路"(w153) -> ()
              n5315 = local write "单选_第65路"(w153) -> ()
              n5316 = local write "单选_第66路"(w153) -> ()
              n5317 = local write "单选_第67路"(w153) -> ()
              n5318 = local write "单选_第68路"(w153) -> ()
              n5319 = local write "单选_第69路"(w153) -> ()
              n5320 = local write "单选_第70路"(w153) -> ()
              n5321 = local write "单选_第72路"(w153) -> ()
              n5322 = local write "单选_第73路"(w153) -> ()
              n5323 = local write "单选_第74路"(w153) -> ()
              n5324 = local write "单选_第75路"(w153) -> ()
              n5325 = local write "单选_第76路"(w153) -> ()
              n5326 = local write "单选_第77路"(w153) -> ()
              n5327 = local write "单选_第78路"(w153) -> ()
              n5328 = local write "单选_第80路"(w153) -> ()
            }
            frame 61 {
              w154 = TRUE
              w155 = FALSE ("单选_第41路")
              n5329 = local write "单选_第1路"(w154) -> ()
              n5330 = local write "单选_第2路"(w154) -> ()
              n5331 = local write "单选_第3路"(w154) -> ()
              n5332 = local write "单选_第4路"(w154) -> ()
              n5333 = local write "单选_第5路"(w154) -> ()
              n5334 = local write "单选_第6路"(w154) -> ()
              n5335 = local write "单选_第7路"(w154) -> ()
              n5336 = local write "单选_第8路"(w154) -> ()
              n5337 = local write "单选_第9路"(w154) -> ()
              n5338 = local write "单选_第10路"(w154) -> ()
              n5339 = local write "单选_第11路"(w154) -> ()
              n5340 = local write "单选_第12路"(w154) -> ()
              n5341 = local write "单选_第13路"(w154) -> ()
              n5342 = local write "单选_第14路"(w154) -> ()
              n5343 = local write "单选_第15路"(w154) -> ()
              n5344 = local write "单选_第16路"(w154) -> ()
              n5345 = local write "单选_第17路"(w154) -> ()
              n5346 = local write "单选_第18路"(w154) -> ()
              n5347 = local write "单选_第19路"(w154) -> ()
              n5348 = local write "单选_第20路"(w154) -> ()
              n5349 = local write "单选_第21路"(w154) -> ()
              n5350 = local write "单选_第22路"(w154) -> ()
              n5351 = local write "单选_第23路"(w154) -> ()
              n5352 = local write "单选_第24路"(w154) -> ()
              n5353 = local write "单选_第25路"(w154) -> ()
              n5354 = local write "单选_第26路"(w154) -> ()
              n5355 = local write "单选_第27路"(w154) -> ()
              n5356 = local write "单选_第28路"(w154) -> ()
              n5357 = local write "单选_第29路"(w154) -> ()
              n5358 = local write "单选_第30路"(w154) -> ()
              n5359 = local write "单选_第31路"(w154) -> ()
              n5360 = local write "单选_第32路"(w154) -> ()
              n5361 = local write "单选_第33路"(w154) -> ()
              n5362 = local write "单选_第34路"(w154) -> ()
              n5363 = local write "单选_第35路"(w154) -> ()
              n5364 = local write "单选_第36路"(w154) -> ()
              n5365 = local write "单选_第37路"(w154) -> ()
              n5366 = local write "单选_第38路"(w154) -> ()
              n5367 = local write "单选_第39路"(w154) -> ()
              n5368 = local write "单选_第40路"(w154) -> ()
              n5369 = local write "单选_第41路"(w154) -> ()
              n5370 = local write "单选_第42路"(w154) -> ()
              n5371 = local write "单选_第43路"(w154) -> ()
              n5372 = local write "单选_第44路"(w154) -> ()
              n5373 = local write "单选_第45路"(w154) -> ()
              n5374 = local write "单选_第46路"(w154) -> ()
              n5375 = local write "单选_第47路"(w154) -> ()
              n5376 = local write "单选_第48路"(w154) -> ()
              n5377 = local write "单选_第49路"(w154) -> ()
              n5378 = local write "单选_第50路"(w154) -> ()
              n5379 = local write "单选_第51路"(w154) -> ()
              n5380 = local write "单选_第52路"(w154) -> ()
              n5381 = local write "单选_第53路"(w154) -> ()
              n5382 = local write "单选_第54路"(w154) -> ()
              n5383 = local write "单选_第55路"(w154) -> ()
              n5384 = local write "单选_第56路"(w154) -> ()
              n5385 = local write "单选_第57路"(w154) -> ()
              n5386 = local write "单选_第58路"(w154) -> ()
              n5387 = local write "单选_第59路"(w154) -> ()
              n5388 = local write "单选_第60路"(w154) -> ()
              n5389 = local write "单选_第61路"(w154) -> ()
              n5390 = local write "单选_第62路"(w155) -> ()
              n5391 = local write "单选_第63路"(w155) -> ()
              n5392 = local write "单选_第64路"(w155) -> ()
              n5393 = local write "单选_第71路"(w155) -> ()
              n5394 = local write "单选_第79路"(w155) -> ()
              n5395 = local write "单选_第65路"(w155) -> ()
              n5396 = local write "单选_第66路"(w155) -> ()
              n5397 = local write "单选_第67路"(w155) -> ()
              n5398 = local write "单选_第68路"(w155) -> ()
              n5399 = local write "单选_第69路"(w155) -> ()
              n5400 = local write "单选_第70路"(w155) -> ()
              n5401 = local write "单选_第72路"(w155) -> ()
              n5402 = local write "单选_第73路"(w155) -> ()
              n5403 = local write "单选_第74路"(w155) -> ()
              n5404 = local write "单选_第75路"(w155) -> ()
              n5405 = local write "单选_第76路"(w155) -> ()
              n5406 = local write "单选_第77路"(w155) -> ()
              n5407 = local write "单选_第78路"(w155) -> ()
              n5408 = local write "单选_第80路"(w155) -> ()
            }
            frame 62 {
              w156 = TRUE
              w157 = FALSE ("单选_第41路")
              n5409 = local write "单选_第1路"(w156) -> ()
              n5410 = local write "单选_第2路"(w156) -> ()
              n5411 = local write "单选_第3路"(w156) -> ()
              n5412 = local write "单选_第4路"(w156) -> ()
              n5413 = local write "单选_第5路"(w156) -> ()
              n5414 = local write "单选_第6路"(w156) -> ()
              n5415 = local write "单选_第7路"(w156) -> ()
              n5416 = local write "单选_第8路"(w156) -> ()
              n5417 = local write "单选_第9路"(w156) -> ()
              n5418 = local write "单选_第10路"(w156) -> ()
              n5419 = local write "单选_第11路"(w156) -> ()
              n5420 = local write "单选_第12路"(w156) -> ()
              n5421 = local write "单选_第13路"(w156) -> ()
              n5422 = local write "单选_第14路"(w156) -> ()
              n5423 = local write "单选_第15路"(w156) -> ()
              n5424 = local write "单选_第16路"(w156) -> ()
              n5425 = local write "单选_第17路"(w156) -> ()
              n5426 = local write "单选_第18路"(w156) -> ()
              n5427 = local write "单选_第19路"(w156) -> ()
              n5428 = local write "单选_第20路"(w156) -> ()
              n5429 = local write "单选_第21路"(w156) -> ()
              n5430 = local write "单选_第22路"(w156) -> ()
              n5431 = local write "单选_第23路"(w156) -> ()
              n5432 = local write "单选_第24路"(w156) -> ()
              n5433 = local write "单选_第25路"(w156) -> ()
              n5434 = local write "单选_第26路"(w156) -> ()
              n5435 = local write "单选_第27路"(w156) -> ()
              n5436 = local write "单选_第28路"(w156) -> ()
              n5437 = local write "单选_第29路"(w156) -> ()
              n5438 = local write "单选_第30路"(w156) -> ()
              n5439 = local write "单选_第31路"(w156) -> ()
              n5440 = local write "单选_第32路"(w156) -> ()
              n5441 = local write "单选_第33路"(w156) -> ()
              n5442 = local write "单选_第34路"(w156) -> ()
              n5443 = local write "单选_第35路"(w156) -> ()
              n5444 = local write "单选_第36路"(w156) -> ()
              n5445 = local write "单选_第37路"(w156) -> ()
              n5446 = local write "单选_第38路"(w156) -> ()
              n5447 = local write "单选_第39路"(w156) -> ()
              n5448 = local write "单选_第40路"(w156) -> ()
              n5449 = local write "单选_第41路"(w156) -> ()
              n5450 = local write "单选_第42路"(w156) -> ()
              n5451 = local write "单选_第43路"(w156) -> ()
              n5452 = local write "单选_第44路"(w156) -> ()
              n5453 = local write "单选_第45路"(w156) -> ()
              n5454 = local write "单选_第46路"(w156) -> ()
